vi "hahahahhahhaGlobal.vi"() -> ()   [LabVIEW 2020]
panel:
  out "Numeric 2":dbl
  in  "Numeric":dbl
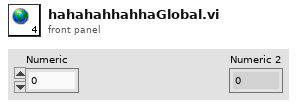
[diagram p1: front panel]
diagram:
